vi "LJM_Close.vi"(8 "error in":errorcluster, 11 "Handle":i32) -> (0 "error out":errorcluster)   [LabVIEW 2025]
uses:
  labjackm.dll
panel:
  # "Calls Close even if error in is true."
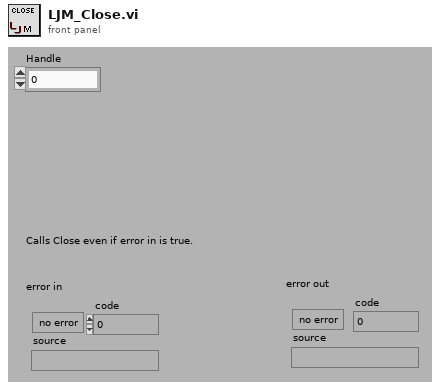
[diagram p1: front panel]
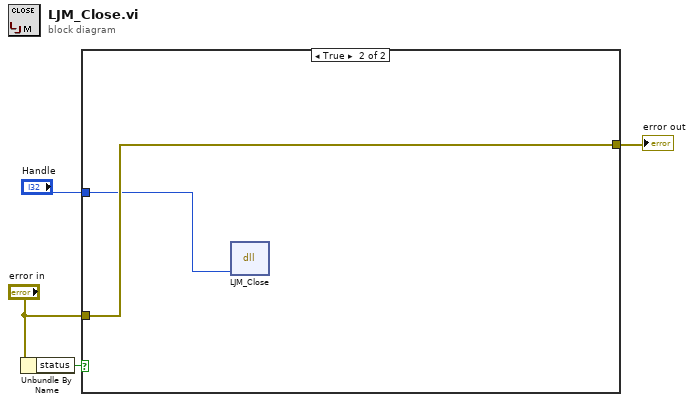
[diagram p0: block diagram]
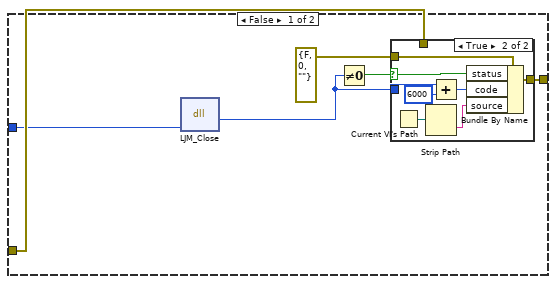
[diagram p2: hidden frame]
diagram:
  n1 = Unbundle By Name("error in") -> ("status"=w3:bool)
  n2 = case shown="True" w3 {
    tunnel: [w7 w21] -> w4
    tunnel: "error in" -> [w6 w21]
    tunnel: "Handle" -> [w5 w20]
    frame False {
      n3 = dll-call lib="labjackm.dll" fn="LJM_Close"("Handle"=w5) -> (w8:i32)  [unwired: 4 in, 2 out]
      n4 = Not Equal To 0?(x=w8) -> (x != 0?=w9:bool)
      n5 = case shown="True" w9 {
        selector: w9 -> [_ w18]
        tunnel: [w11 w19] -> w7
        tunnel: errorcluster {"status"=FALSE, "code"=0, "source"=""} ("error IO") -> [_ w17]
        tunnel: w8 -> [_ w13]
        tunnel: w6 -> [w11 _]
        frame False {
        }
        frame True {
          n6 = Current VI's Path() -> (path=w15:path)
          n7 = Strip Path(path=w15) -> (name=w16:string)  [unwired: 1 out]
          n8 = Add(x=w13, y=6000) -> (x+y=w14:i32)
          n9 = Bundle By Name(cluster=w17, "status"=w18, "code"=w14, "source"=w16) -> (w19:errorcluster)
        }
      }
    }
    frame True {
      n10 = dll-call lib="labjackm.dll" fn="LJM_Close"("Handle"=w20) -> ()  [unwired: 5 in, 2 out]
    }
  }
  "error out" <- w4
